vi "Write Alarm Limits - Low Warning Severity.vi"(8 "error in (no error)":errorcluster, 10 "low warning severity":T1, 11 "NT Scalar (Numeric) in":refnum<class "NT Scalar (Numeric).lvclass">) -> (0 "error out":errorcluster, 3 "NT Scalar (Numeric) out":refnum<class "NT Scalar (Numeric).lvclass">)   [LabVIEW 2020, in "PV Access.lvlib" / "PV Data.lvlib" / "NT Scalar (Numeric).lvclass"]
uses:
  NT Scalar (Numeric).lvclass
  NT Scalar (Numeric).lvclass/NT Scalar (Numeric).ctl
  Alarm Severity.ctl
  PV Data.lvlib
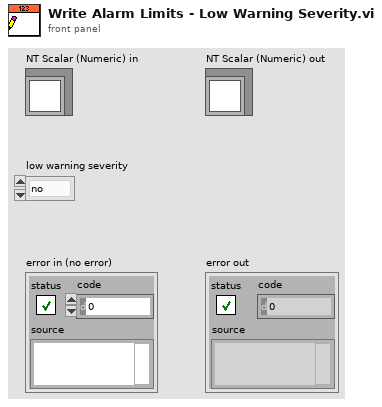
[diagram p1: front panel]
types:
  T1 = typedef "PV Access.lvlib/PV Data.lvlib/Alarm Severity.ctl" = enum32{"no", "minor", "major", "record", "invalid", "undefined"}
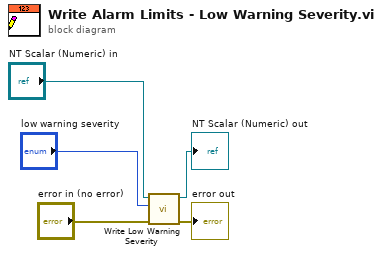
[diagram p0: block diagram]
diagram:
  n1 = call-dynamic "Write Low Warning Severity.vi"("error in"="error in (no error)", "low warning severity"="low warning severity", "Has Alarm Limits in"="NT Scalar (Numeric) in") -> ("error out"=→"error out":errorcluster, "Has Alarm Limits out"=→"NT Scalar (Numeric) out":refnum<class "NT Scalar (Numeric).lvclass">)  [unwired: 7 in]
